vi "Test Method.vi"(11 "Test Case In":refnum<class "Test&Case.lvclass">) -> (0 "error out":errorcluster, 3 "Test Case Out":refnum<class "Test&Case.lvclass">)   [LabVIEW 2020, in "Test&Case.lvclass"]
uses:
  Test&Case.lvclass
  C:/git/astemes-lunit/source/Core/LUnit Test Case/LUnit Test Case.lvclass
  source/LUnit Test Case.lvclass/LUnit Test Case.ctl
  108a9ea9-4cba-4065-a0e2-59bd5e3a3d12.vi
  source/Core/LUnit Test Case/Private/Append Pass Result.vi
  source/Core/LUnit Test Case/Private/Append Fail Result.vi
  108a9ea9-4cba-4065-a0e2-59bd5e3a3d12.vi/9c5d11cd-9439-4240-a1ee-d9baace9c924.vi
  source/Core/LUnit Test Case/Private/Run In UI.vi
  <vilib>/Utility/error.llb/Clear Errors.vi
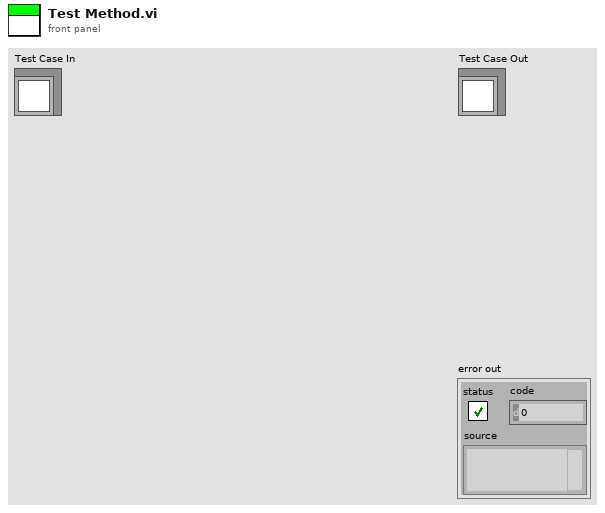
[diagram p1: front panel]
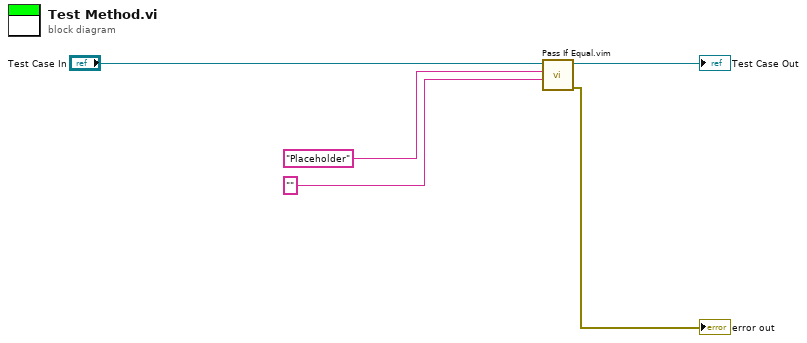
[diagram p0: block diagram]
diagram:
  n1 = call "Pass If Equal.vim"("Actual"="", "Expected"="Placeholder", "LUnit Test Case In"="Test Case In") -> ("error out"=→"error out":errorcluster, "LUnit Test Case Out"=→"Test Case Out":refnum<class "Test&Case.lvclass">)  [unwired: 7 in]
